vi "Main.vi"(8 "error in":errorcluster, 11 "Scope Simulator in":refnum<class "Scope Simulator.lvclass">) -> (0 "error out":errorcluster, 3 "Scope Simulator out":refnum<class "Scope Simulator.lvclass">)   [LabVIEW 2019, in "Scope Simulator.lvclass"]
doc: "The <b>Queued Message Handler</b> of the Worker that owns this VI."
uses:
  Scope Simulator.lvclass
  rsp_Scope Status.ctl
  Initialization Data.ctl
  Response Cases.ctl
  <vilib>/addons/_Workers/Library/Case Label.ctl
  Scope Simulator.lvclass/Scope Simulator.ctl
  rql_Generate Waveform.ctl
  rsp_Generated Waveform.ctl
  rqp_Run Scope.ctl
  rwr_Get Device Info.ctl
  rwr_Get Device Info Reply.ctl
  rqp_Scope Configuration.ctl
  rwr_Get Scope State.ctl
  rwr_Get Scope State Reply.ctl
  <vilib>/addons/_Workers/Library/Workers.lvlib
panel:
  in  "Select":u16(ring) items=["Sine", "Square", "Triangle", "Sawtooth", "DC"]
  out "Scope Configuration":T1
  out "Acquisitions":i32
  out "Scope State":T2
  out "Waveform":dynamicdata(graph) caption="Sine"
  in  "Frequency":dbl(slide)=49.735 min=0.0 max=49.735 scale=0.0..50.0
  in  "Amplitude":dbl(slide)=5.0 min=0.0 max=5.0 scale=0.0..5.0
  in  "Scope Device Info":cluster{"device":string, "product_type":string}={"device"="NI Scope", "product_type"="Simulated"}
  # "Generic Scope Simulator"
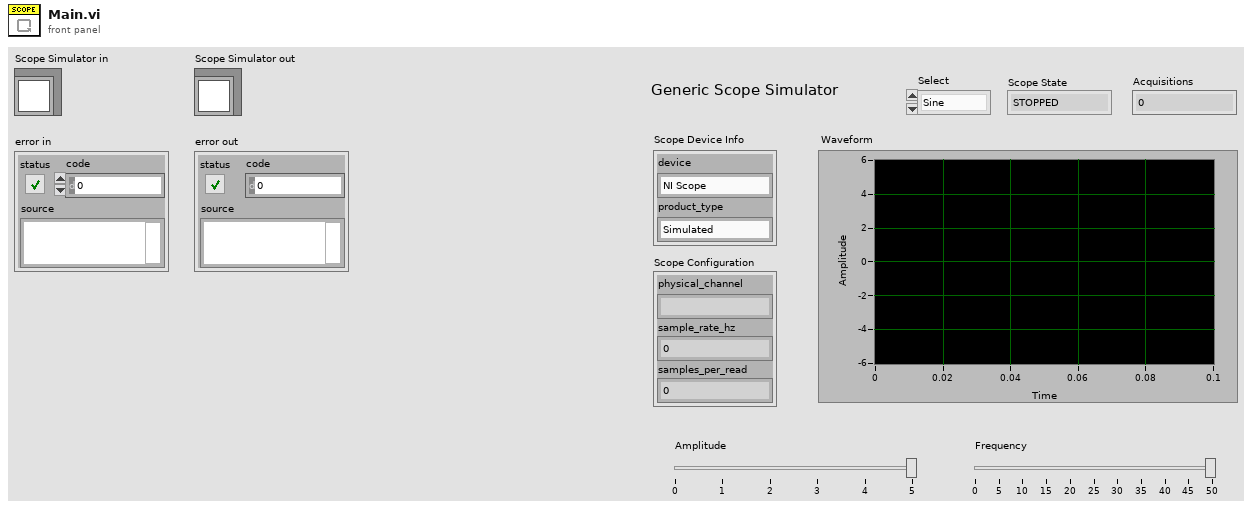
[diagram p1: front panel]
types:
  T1 = cluster{"physical_channel":string, "sample_rate_hz":dbl, "samples_per_read":i32}
  T2 = typedef "Scope Simulator.lvclass/rsp_Scope Status.ctl" = enum32{"STOPPED", "RUNNING", "ERROR"}
  T3 = typedef "Scope Simulator.lvclass/Initialization Data.ctl" = cluster{"Response Cases":T4}
  T4 = typedef "Scope Simulator.lvclass/Response Cases.ctl" = cluster{"Generated Waveform":T5, "Scope Status":T5}
  T5 = typedef "Workers.lvlib/Case Label.ctl" = string
  T6 = typedef "Scope Simulator.lvclass/rql_Generate Waveform.ctl" = cluster{"String":string}
  T7 = typedef "Scope Simulator.lvclass/rsp_Generated Waveform.ctl" = cluster{"y":dbl[], "Acquisitions":i32}
  T8 = typedef "Scope Simulator.lvclass/rqp_Run Scope.ctl" = cluster{"Run Scope ?":bool}
  T9 = typedef "Scope Simulator.lvclass/rwr_Get Device Info Reply.ctl" = cluster{"device":string, "product_type":string}
  T10 = typedef "Scope Simulator.lvclass/rwr_Get Device Info.ctl" = cluster{"String":string}
  T11 = typedef "Scope Simulator.lvclass/rqp_Scope Configuration.ctl" = cluster{"physical_channel":string, "sample_rate_hz":dbl, "samples_per_read":i32}
  T12 = typedef "Scope Simulator.lvclass/rwr_Get Scope State Reply.ctl" = cluster{"Scope State":T2}
  T13 = typedef "Scope Simulator.lvclass/rwr_Get Scope State.ctl" = cluster{"String":string}
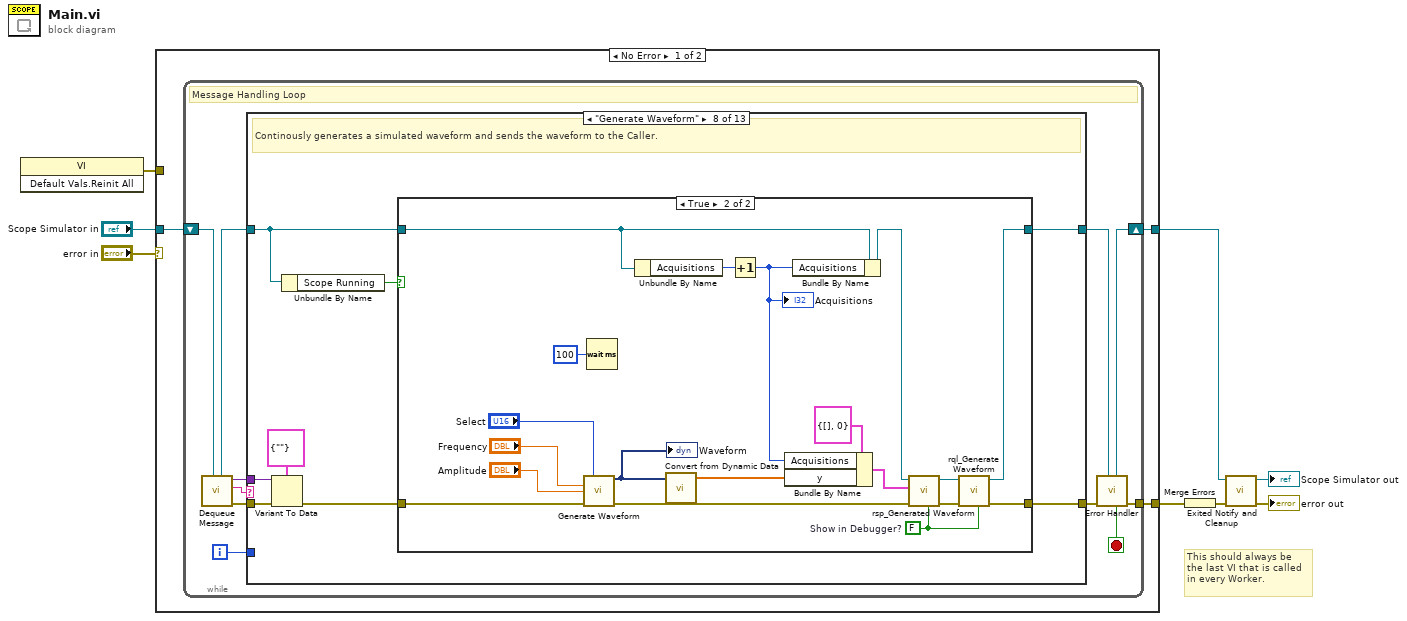
[diagram p0: block diagram]
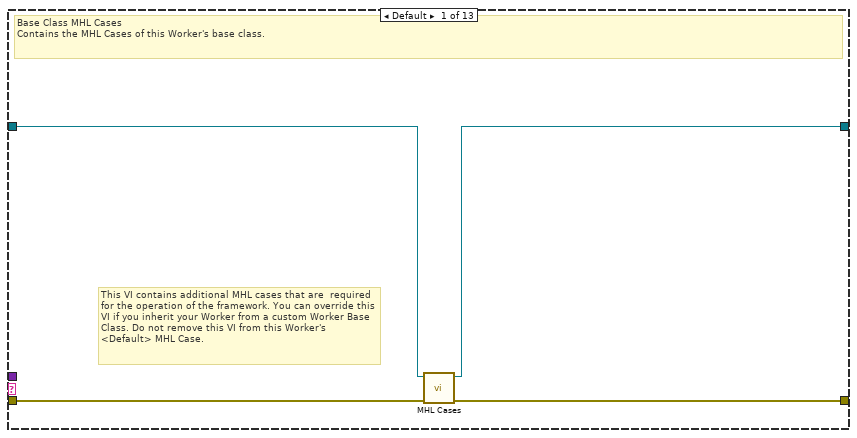
[diagram p2: hidden frame]
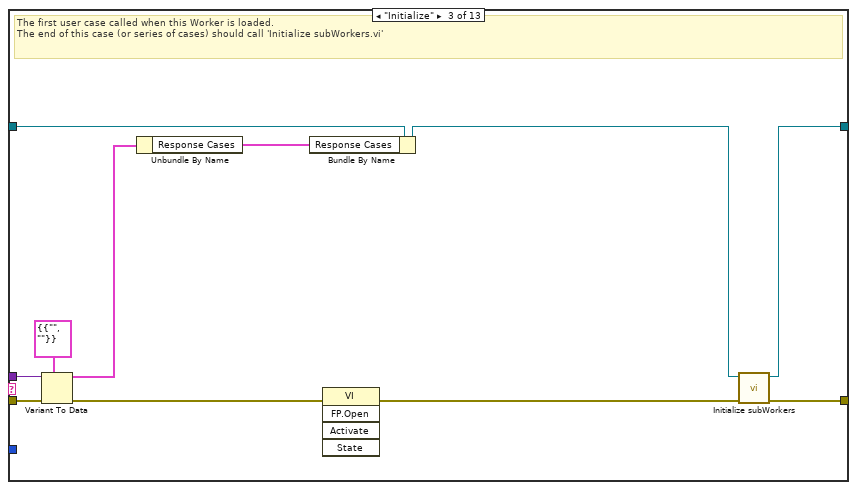
[diagram p4: hidden frame]
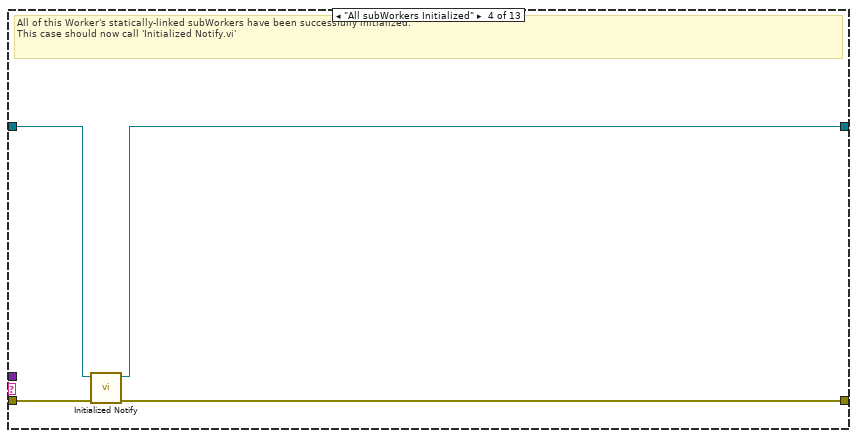
[diagram p5: hidden frame]
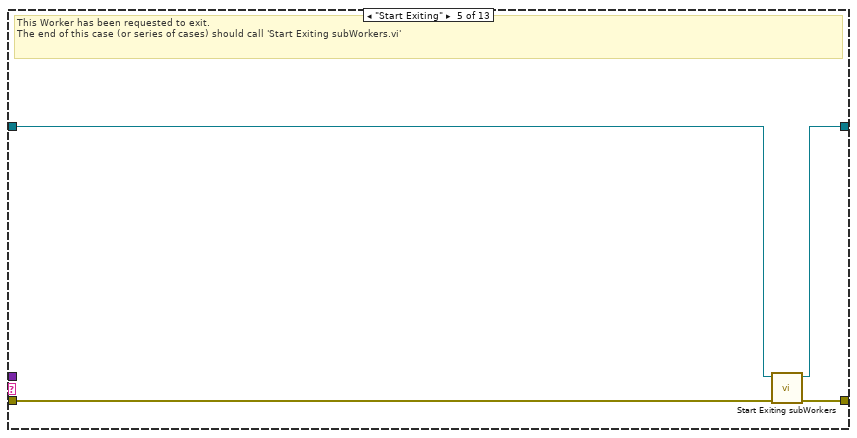
[diagram p6: hidden frame]
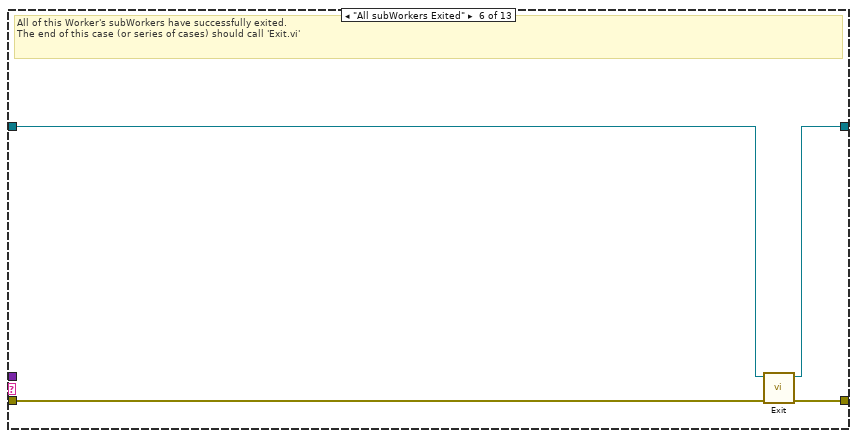
[diagram p7: hidden frame]
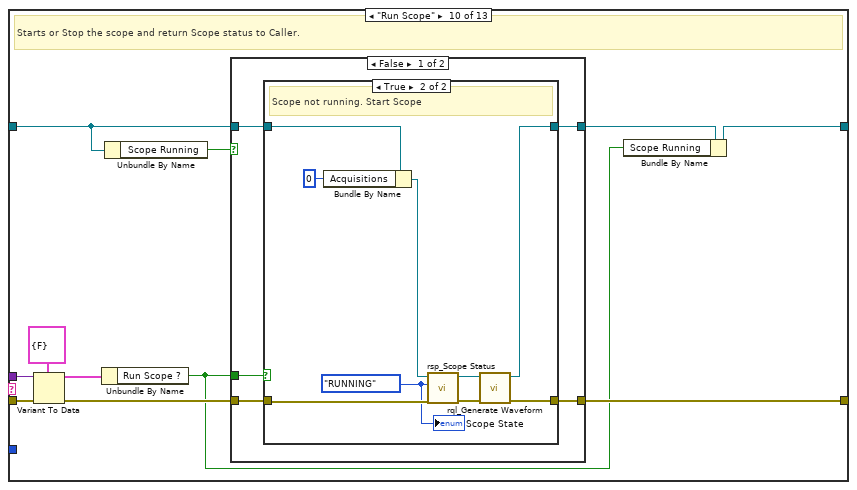
[diagram p11: hidden frame]
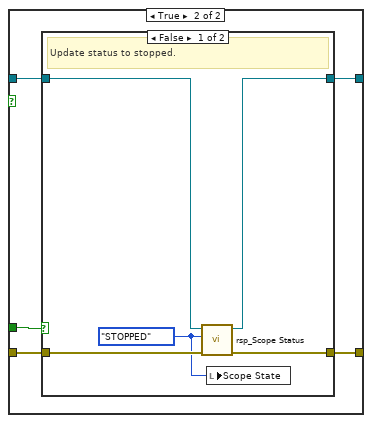
[diagram p13: hidden frame]
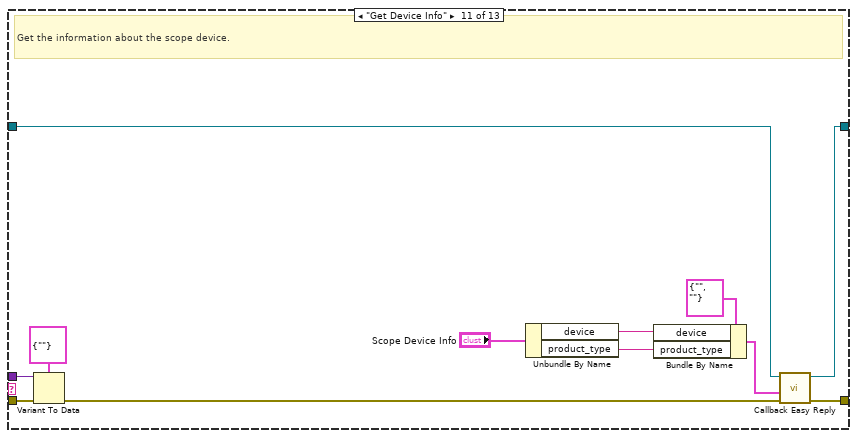
[diagram p15: hidden frame]
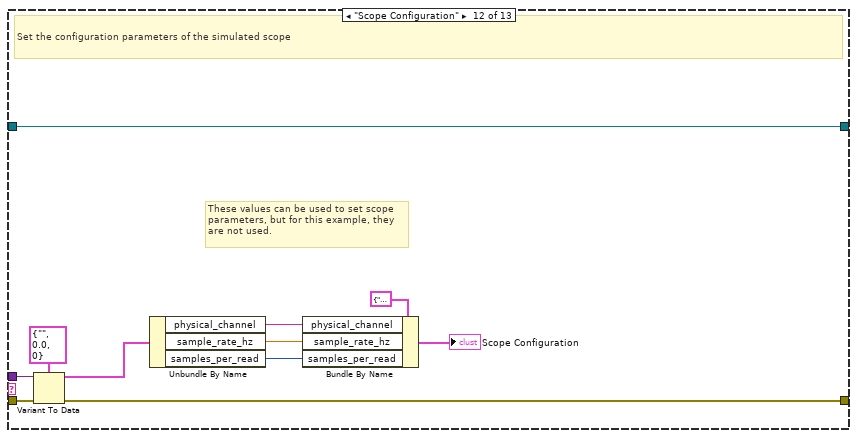
[diagram p16: hidden frame]
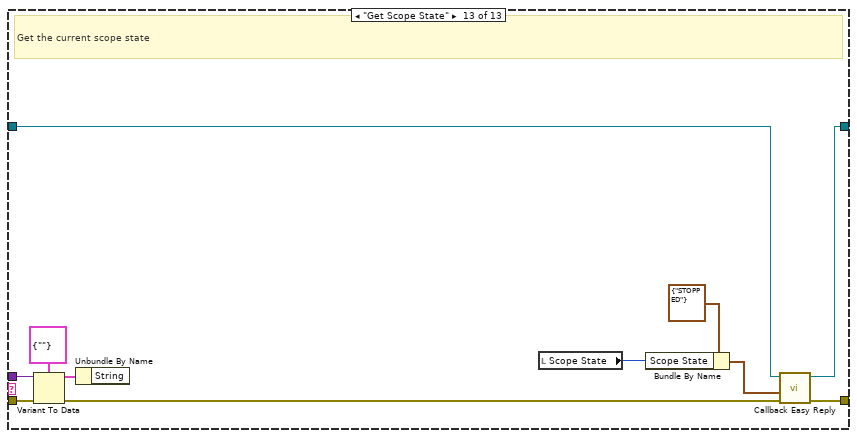
[diagram p17: hidden frame]
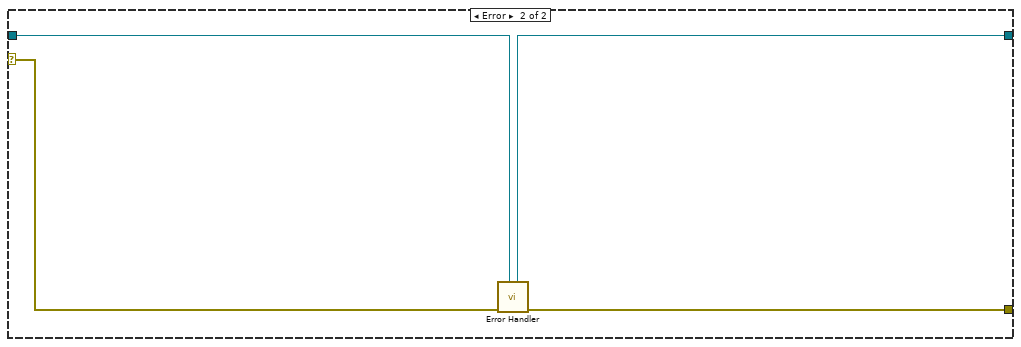
[diagram p18: hidden frame]
diagram:
  # "This should always be the last VI that is called in every Worker."
  n1 = invoke class="VI" method="Default Vals.Reinit All"() -> (error out=w3:errorcluster)  [unwired: 3 in, 2 out]
  n2 = case shown="No Error" "error in" {
    tunnel: "Scope Simulator in" -> [w11 w159]
    tunnel: [w9 w160] -> w6
    tunnel: [w10 w158] -> w7
    selector: "error in" -> [_ w161]
    tunnel: w3 -> [_ _]
    frame No Error {
      n3 = while {
        shift-right: [w20] -> w10
        shift-left: w11 -> [w22]
        tunnel: [w21] -> w9
        i -> [w13]
        stop <- w14 stop-if-true
        # "Message Handling Loop"
        n4 = call-dynamic "Dequeue Message.vi"("Worker"=w22) -> ("error out"=w19:errorcluster, "Case out"=w15:string, "Data out"=w12:variant, "Worker out"=w17:refnum<class "Scope Simulator.lvclass">)  [unwired: 6 in, 1 out]
        n5 = case "Worker MHL Case Structure (DO NOT CHANGE LABEL NAME)" shown="\"Generate Waveform\"" w15 {
          tunnel: w19 -> [w26 w27 w37 w41 w44 w51 w53 w61 w84 w95 w135 w145 w157]
          tunnel: [w25 w27 w39 w40 w47 w50 w53 w57 w84 w90 w131 w144 w152] -> w18
          tunnel: w17 -> [w24 w28 w36 w43 w45 w49 w52 w55 w83 w88 w129 w146 w150]
          tunnel: [w23 w28 w38 w42 w46 w48 w52 w56 w83 w86 w130 w146 w151] -> w16
          tunnel: w13 -> [_ _ _ _ _ _ _ _ _ _ _ _ _]
          tunnel: w12 -> [_ _ w35 _ _ _ _ w58 _ w92 w132 w142 w154]
          frame Default {
            # "This VI contains additional MHL cases that are  required for the operation of the framework. You can override this VI if you inherit your Worker from a custom Worker Base Class. Do not remove this VI from this Worker's <Default> MHL Case."
            # "Base Class MHL Cases\nContains the MHL Cases of this Worker's base class."
            n6 = call-dynamic "MHL Cases.vi"("error in"=w26, "Worker in"=w24) -> ("error out"=w25:errorcluster, "Worker out"=w23:refnum<class "Scope Simulator.lvclass">)  [unwired: 8 in]
          }
          frame "------------ FRAMEWORK CASES -----------" {
            # "Start of Workers Framework Cases"
          }
          frame "Initialize" {
            # "The first user case called when this Worker is loaded.\nThe end of this case (or series of cases) should call 'Initialize subWorkers.vi'"
            n7 = Variant To Data(error in=w37, type=T3 {"Response Cases"={"Generated Waveform"="", "Scope Status"=""}} ("Initialization Data"), Variant=w35) -> (data=w33:T3, error out=w30:errorcluster)
            n8 = Unbundle By Name(w33) -> ("Response Cases"=w32:T4)
            n9 = Bundle By Name(cluster=w36, "Response Cases"=w32) -> (w34:refnum<class "Scope Simulator.lvclass">)
            n10 = invoke class="VI" method="FP.Open"(error in=w30) -> (error out=w29:errorcluster)  [unwired: 4 in, 4 out]
            n11 = call-dynamic "Initialize subWorkers.vi"("error in"=w29, "Worker"=w34) -> ("error out"=w39:errorcluster, "dup Worker out"=w38:refnum<class "Scope Simulator.lvclass">)  [unwired: 8 in]
          }
          frame "All subWorkers Initialized" {
            # "All of this Worker's statically-linked subWorkers have been successfully initialized.\nThis case should now call 'Initialized Notify.vi'"
            n12 = call-dynamic "Initialized Notify.vi"("error in"=w41, "Worker"=w43) -> ("error out"=w40:errorcluster, "dup Worker out"=w42:refnum<class "Scope Simulator.lvclass">)  [unwired: 8 in]
          }
          frame "Start Exiting" {
            # "This Worker has been requested to exit. \nThe end of this case (or series of cases) should call 'Start Exiting subWorkers.vi'"
            n13 = call-dynamic "Start Exiting subWorkers.vi"("error_in"=w44, "Worker"=w45) -> ("error out"=w47:errorcluster, "dup Worker out"=w46:refnum<class "Scope Simulator.lvclass">)  [unwired: 8 in]
          }
          frame "All subWorkers Exited" {
            # "All of this Worker's subWorkers have successfully exited. \nThe end of this case (or series of cases) should call 'Exit.vi'"
            n14 = call-dynamic "Exit.vi"("error_in"=w51, "Worker"=w49) -> ("error out"=w50:errorcluster, "dup Worker out"=w48:refnum<class "Scope Simulator.lvclass">)  [unwired: 8 in]
          }
          frame "------------- LOCAL API CASES -------------" {
            # "Start of Workers Local API Cases"
          }
          frame "Generate Waveform" {
            # "Continously generates a simulated waveform and sends the waveform to the Caller."
            n15 = Variant To Data(error in=w61, type=T6 {"String"=""} ("Data"), Variant=w58) -> (error out=w60:errorcluster)  [unwired: 1 out]
            n16 = Unbundle By Name(w55) -> ("Scope Running"=w54:bool)
            n17 = case shown="True" w54 {
              tunnel: w60 -> [w62 w78]
              tunnel: [w62 w76] -> w57
              tunnel: w55 -> [w63 w71]
              tunnel: [w63 w74] -> w56
              frame False {
              }
              frame True {
                w73 = FALSE  # Show in Debugger?
                n18 = call "Generate Waveform.vi"("Waveform"="Select", "Frequency"="Frequency", "Amplitude"="Amplitude", "error in (no error)"=w78) -> ("Sine"=w64:dynamicdata, "error out"=w77:errorcluster)  [unwired: 10 in]
                "Waveform" <- w64
                n19 = Wait (ms)(milliseconds to wait=u32 100) -> ()  [unwired: 1 out]
                n20 = Unbundle By Name(w71) -> ("Acquisitions"=w70:i32)
                n21 = call "Convert from Dynamic Data"("Dynamic Data Type"=w64) -> ("Array"=w79:dbl[])  [unwired: 3 in]
                n22 = Increment(x=w70) -> (x+1=w69:i32)
                "Acquisitions" <- w69
                n23 = Bundle By Name(cluster=T7 {"y"=[], "Acquisitions"=0} ("Data in"), "Acquisitions"=w69, "y"=w79) -> (w80:T7)
                n24 = Bundle By Name(cluster=w71, "Acquisitions"=w69) -> (w72:refnum<class "Scope Simulator.lvclass">)
                n25 = call "rsp_Generated Waveform.vi"("Show in Debugger?"=w73, "error in"=w77, "Data in"=w80, "Scope Simulator in"=w72) -> ("error out"=w82:errorcluster, "dup Scope Simulator out"=w75:refnum<class "Scope Simulator.lvclass">)  [unwired: 6 in]
                n26 = call "rql_Generate Waveform.vi"("Show in Debugger?"=w73, "error in"=w82, "Scope Simulator in"=w75) -> ("error out"=w76:errorcluster, "dup Scope Simulator out"=w74:refnum<class "Scope Simulator.lvclass">)  [unwired: 7 in]
              }
            }
          }
          frame "------------- PUBLIC API CASES -------------" {
            # "Start of Workers Public API Cases"
          }
          frame "Run Scope" {
            # "Starts or Stop the scope and return Scope status to Caller."
            n27 = Variant To Data(error in=w95, type=T8 {"Run Scope ?"=FALSE} ("Data"), Variant=w92) -> (data=w91:T8, error out=w94:errorcluster)
            n28 = Unbundle By Name(w91) -> ("Run Scope ?"=w85:bool)
            n29 = Unbundle By Name(w88) -> ("Scope Running"=w87:bool)
            n30 = case shown="False" w87 {
              tunnel: w94 -> [w100 w116]
              tunnel: [w99 w115] -> w90
              tunnel: [w98 w114] -> w89
              tunnel: w88 -> [w97 w113]
              tunnel: w85 -> [w96 w112]
              frame False {
                n31 = case shown="True" w96 {
                  tunnel: w100 -> [w101 w111]
                  tunnel: [w101 w110] -> w99
                  tunnel: w97 -> [w102 w104]
                  tunnel: [w102 w109] -> w98
                  frame False {
                    # "Scope already stopped. Nothing to do."
                  }
                  frame True {
                    w103 = rsp_Scope_Status."RUNNING" ("Data in")
                    # "Scope not running. Start Scope"
                    n32 = Bundle By Name(cluster=w104, "Acquisitions"=0) -> (w105:refnum<class "Scope Simulator.lvclass">)
                    n33 = call "rsp_Scope Status.vi"("error in"=w111, "Data in"=w103, "Scope Simulator in"=w105) -> ("error out"=w108:errorcluster, "dup Scope Simulator out"=w107:refnum<class "Scope Simulator.lvclass">)  [unwired: 7 in]
                    n34 = call "rql_Generate Waveform.vi"("error in"=w108, "Scope Simulator in"=w107) -> ("error out"=w110:errorcluster, "dup Scope Simulator out"=w109:refnum<class "Scope Simulator.lvclass">)  [unwired: 8 in]
                    "Scope State" <- w103
                  }
                }
              }
              frame True {
                n35 = case shown="False" w112 {
                  tunnel: w116 -> [w121 w123]
                  tunnel: [w120 w123] -> w115
                  tunnel: w113 -> [w117 w122]
                  tunnel: [w119 w122] -> w114
                  frame False {
                    w118 = rsp_Scope_Status."STOPPED" ("Data in")
                    # "Update status to stopped."
                    n36 = call "rsp_Scope Status.vi"("error in"=w121, "Data in"=w118, "Scope Simulator in"=w117) -> ("error out"=w120:errorcluster, "dup Scope Simulator out"=w119:refnum<class "Scope Simulator.lvclass">)  [unwired: 7 in]
                    n37 = local write "Scope State"(w118) -> ()
                  }
                  frame True {
                    # "Scope Running. Nothing to do"
                  }
                }
              }
            }
            n38 = Bundle By Name(cluster=w89, "Scope Running"=w85) -> (w86:refnum<class "Scope Simulator.lvclass">)
          }
          frame "Get Device Info" {
            # "Get the information about the scope device."
            n39 = Variant To Data(error in=w135, type=T10 {"String"=""} ("Data"), Variant=w132) -> (error out=w134:errorcluster)  [unwired: 1 out]
            n40 = Unbundle By Name("Scope Device Info") -> ("device"=w125:string, "product_type"=w124:string)
            n41 = Bundle By Name(cluster=T9 {"device"="", "product_type"=""} ("Reply Data"), "device"=w125, "product_type"=w124) -> (w127:T9)
            n42 = call-dynamic "Callback Easy Reply.vi"("error in"=w134, "Data"=w127, "Worker"=w129) -> ("error out"=w131:errorcluster, "dup Worker out"=w130:refnum<class "Scope Simulator.lvclass">)  [unwired: 7 in]
          }
          frame "Scope Configuration" {
            # "These values can be used to set scope\nparameters, but for this example, they\nare not used."
            # "Set the configuration parameters of the simulated scope"
            n43 = Variant To Data(error in=w145, type=T11 {"physical_channel"="", "sample_rate_hz"=0.0, "samples_per_read"=0} ("Data"), Variant=w142) -> (data=w141:T11, error out=w144:errorcluster)
            n44 = Unbundle By Name(w141) -> ("physical_channel"=w138:string, "sample_rate_hz"=w136:dbl, "samples_per_read"=w137:i32)
            n45 = Bundle By Name(cluster=T1 {"physical_channel"="", "sample_rate_hz"=0.0, "samples_per_read"=0} ("Scope Configuration"), "physical_channel"=w138, "sample_rate_hz"=w136, "samples_per_read"=w137) -> (→"Scope Configuration":T1)
          }
          frame "Get Scope State" {
            # "Get the current scope state"
            n46 = Variant To Data(error in=w157, type=T13 {"String"=""} ("Data"), Variant=w154) -> (data=w153:T13, error out=w156:errorcluster)
            n47 = Unbundle By Name(w153) -> ()  [unwired: 1 out]
            n48 = local read "Scope State"() -> (w147:T2)
            n49 = Bundle By Name(cluster=T12 {"Scope State"=enum."STOPPED"} ("Reply Data"), "Scope State"=w147) -> (w149:T12)
            n50 = call-dynamic "Callback Easy Reply.vi"("error in"=w156, "Data"=w149, "Worker"=w150) -> ("error out"=w152:errorcluster, "dup Worker out"=w151:refnum<class "Scope Simulator.lvclass">)  [unwired: 7 in]
          }
        }
        n51 = call-dynamic "Error Handler.vi"("Worker"=w16, "error_in"=w18) -> ("error out"=w21:errorcluster, "Stop Loop"=w14:bool, "Worker out"=w20:refnum<class "Scope Simulator.lvclass">)  [unwired: 7 in]
      }
    }
    frame Error {
      n52 = call-dynamic "Error Handler.vi"("Worker"=w159, "error_in"=w161) -> ("error out"=w160:errorcluster, "Worker out"=w158:refnum<class "Scope Simulator.lvclass">)  [unwired: 7 in, 1 out]
    }
  }
  n53 = Merge Errors(w6) -> (w8:errorcluster)
  n54 = call-dynamic "Exited Notify and Cleanup.vi"("error_in"=w8, "Worker"=w7) -> ("error out"=→"error out":errorcluster, "dup Worker out"=→"Scope Simulator out":refnum<class "Scope Simulator.lvclass">)  [unwired: 8 in]
